vi "Keyence_读取多个寄存器数据.vi"(0 "Keyence ID In":refnum<k5>, 1 "Delay Time (s)":dbl=1.0 caption="延迟时间(s)", 5 "起始软元件编号":string, 9 "读取个数":string, 11 "错误输入（无错误）":errorcluster) -> (4 "Keyence ID Out":refnum<k5>, 6 "全部数据输出":string, 8 "结果数组":string[](array[string]), 15 "错误输出":errorcluster)   [LabVIEW 2017]
panel:
  out "连接的字符串":string
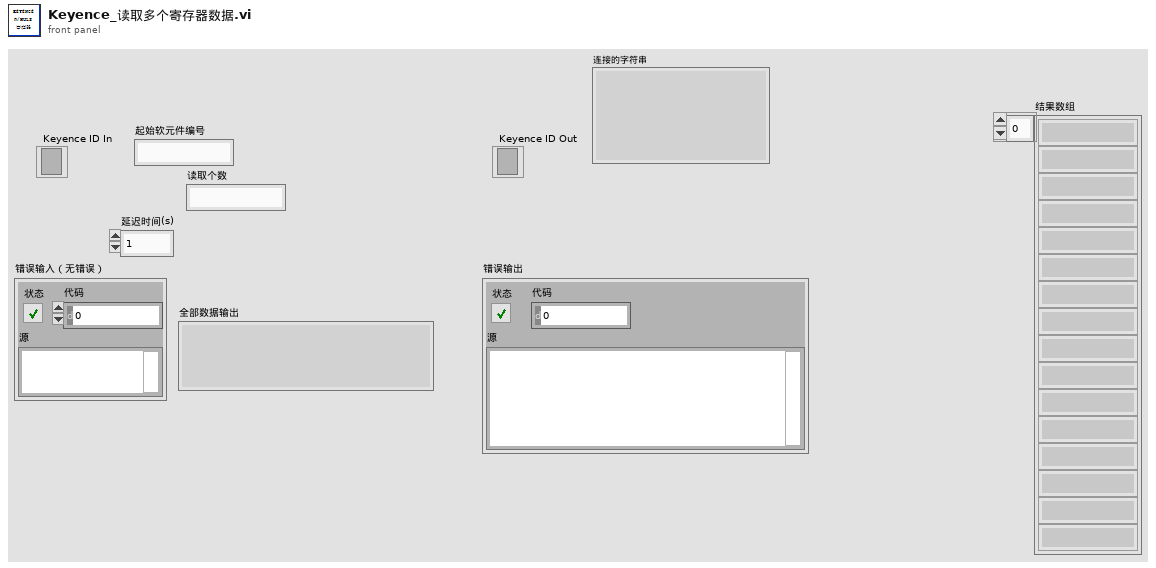
[diagram p1: front panel]
types:
  T1 = enum16{"Standard", "Buffered", "CRLF", "Immediate"}
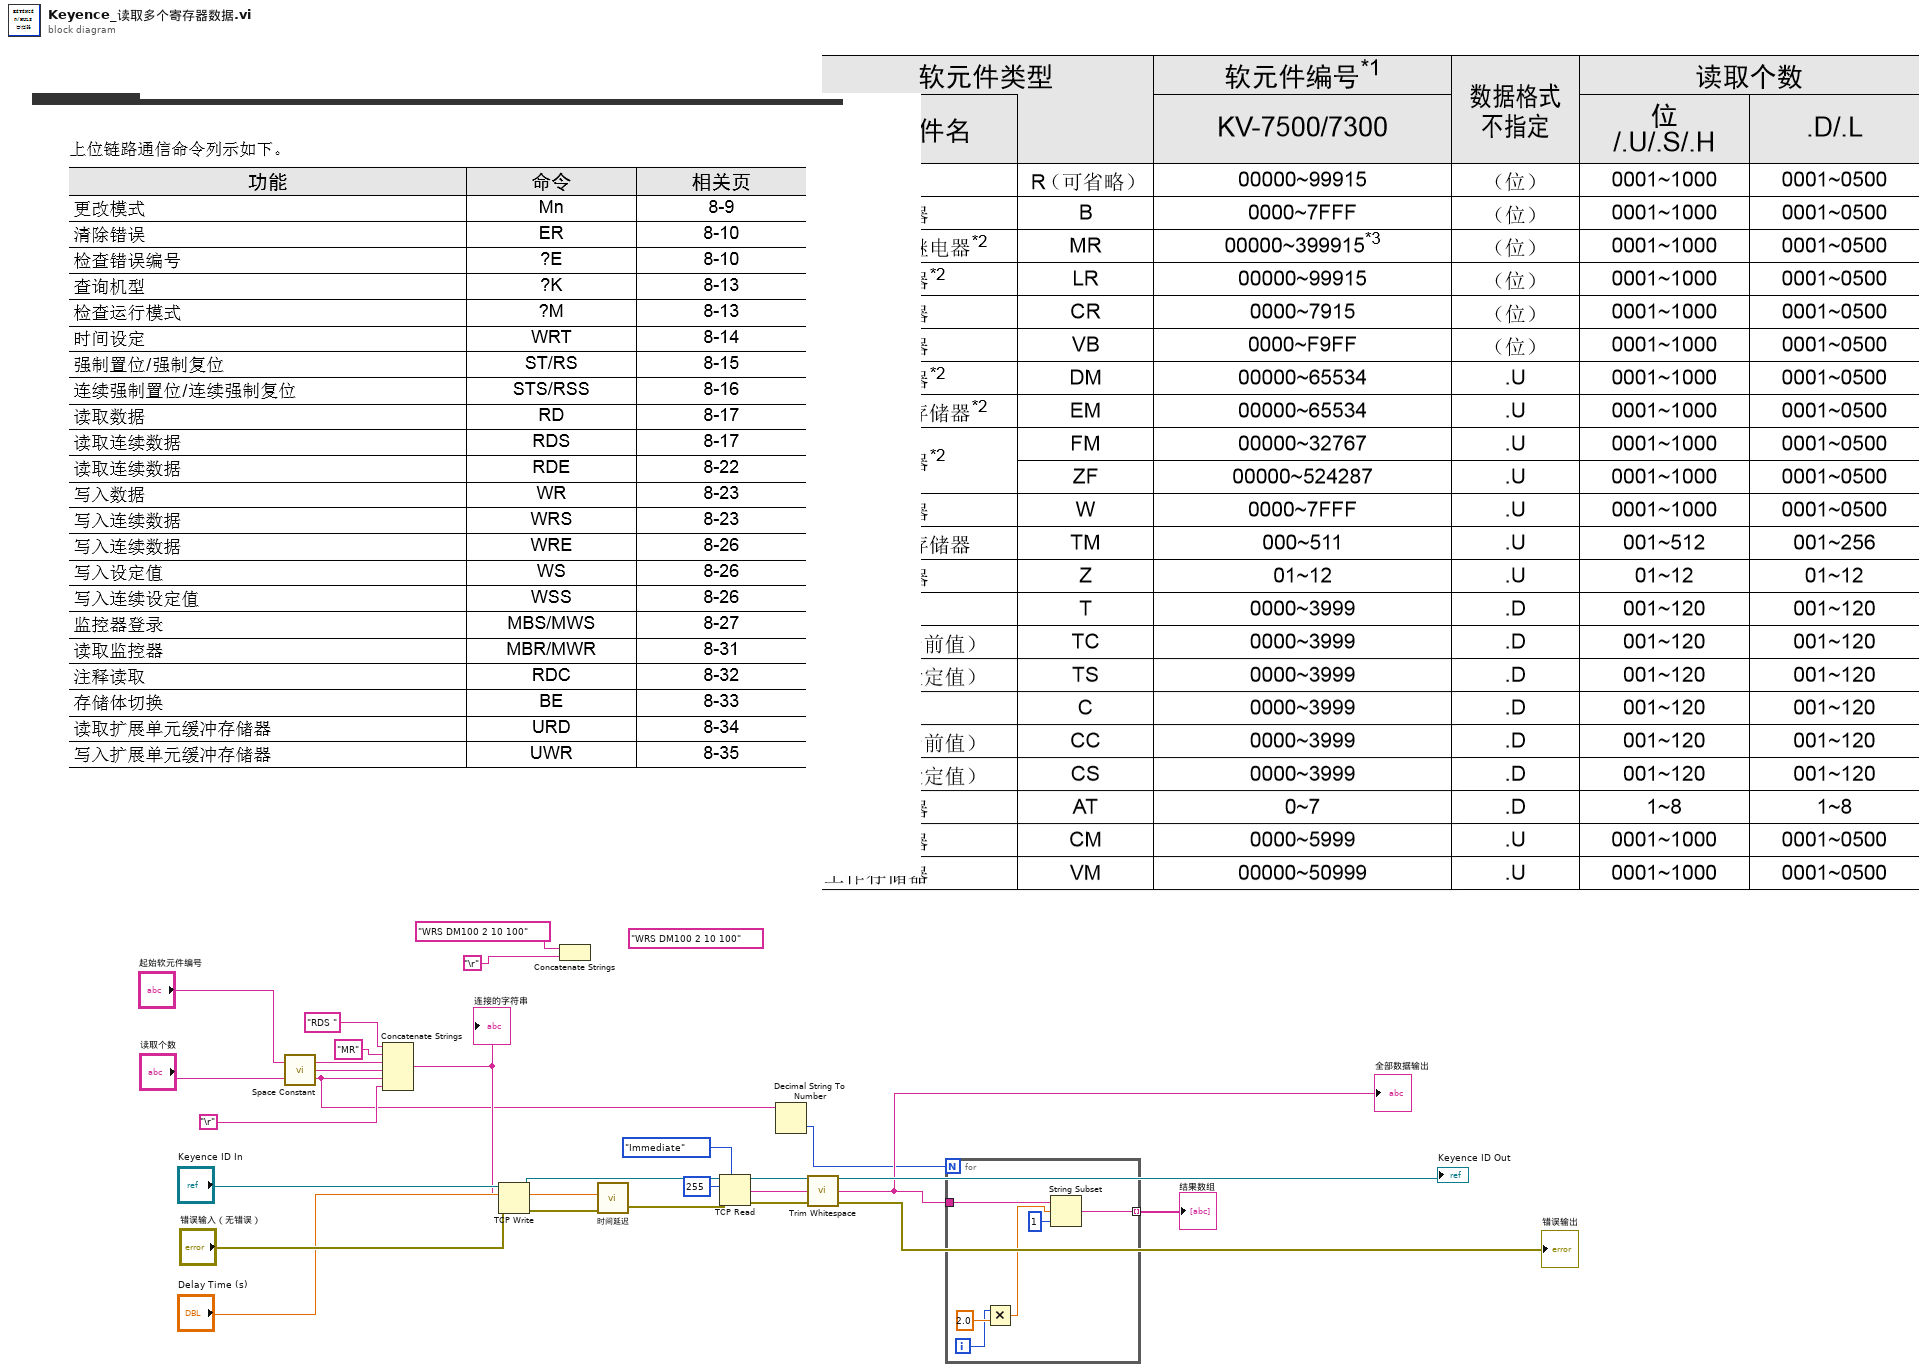
[diagram p0: block diagram]
diagram:
  (unwired) "WRS DM100 2 10 100"
  n1 = call <vilib>:"Space Constant.vi"() -> ("String"=w10:string)
  n2 = Concatenate Strings("RDS ", "MR" ("字符串"), "起始软元件编号", w10, "读取个数", "\r") -> (w8:string)
  "连接的字符串" <- w8
  n3 = TCP Write(connection ID="Keyence ID In", data in=w8, error in (no error)="错误输入（无错误）") -> (connection ID out=w21:refnum<k5>, error out=w20:errorcluster)  [unwired: 1 in, 1 out]
  n4 = Concatenate Strings("WRS DM100 2 10 100", "\r") -> ()  [unwired: 1 out]
  n5 = call "时间延迟"("error in (no error)"=w20, "Delay Time (s)"="Delay Time (s)") -> ("error out"=w15:errorcluster)  [unwired: 9 in]
  n6 = TCP Read(connection ID=w21, bytes to read=255 ("读取的字节"), error in (no error)=w15, 7:T1."Immediate" ("模式（标准）")) -> (connection ID out=→"Keyence ID Out":refnum<k5>, data out=w6:string, error out=→"错误输出":errorcluster)  [unwired: 1 in]
  n7 = Decimal String To Number(string="读取个数") -> (number=w3:i32)  [unwired: 2 in, 1 out]
  n8 = call <vilib>:"Trim Whitespace.vi"("string"=w6) -> ("trimmed string"=w5:string)  [unwired: 1 in]
  "全部数据输出" <- w5
  n9 = for {
    N: w3 -> [_]
    tunnel: w5 -> [w29]
    tunnel: [w24] -> w2 mode=indexing
    i -> [w26]
    n10 = Multiply(x=w26, y=2.0) -> (x*y=w25:dbl)
    n11 = String Subset(string=w29, offset (0)=w25, length (rest)=1 ("长度（剩余）")) -> (substring=w24:string)
  }
  "结果数组" <- w2
